vi "Close Session.vi"(8 "error in":errorcluster, 11 "session":refnum<class "Session.lvclass">) -> (0 "error out":errorcluster)   [LabVIEW 2024, in "lib_NI_Advanced HTTP Client.lvlib" / "Session.lvclass"]
doc: "Closes the HTTP client session and deletes all stored cookies, authentication credentials, and HTTP headers associated with the client session. This VI also terminates all HTTP connections and logs out of any authentication, if applicable."
uses:
  Session.lvclass
  Session.lvclass/Session.ctl
  lvwebclient_64.dll
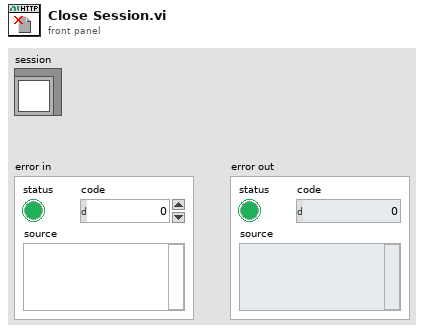
[diagram p1: front panel]
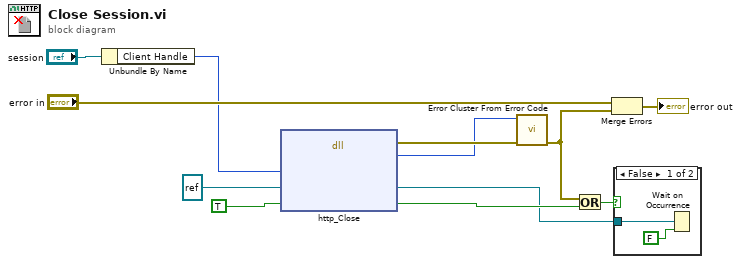
[diagram p0: block diagram]
diagram:
  n1 = Unbundle By Name("session") -> ("Client Handle"=w9:u32)
  n2 = dll-call lib="C:/Program Files/National Instruments/LabVIEW 2024/vi.lib/NI/Advanced HTTP Client/lvwebclient_*.*" fn="http_Close"("handle"=w9, "completeOccurrence"=refnum<k4> refnum ("occurrence"), "closed"=TRUE) -> (error out=w12:errorcluster, "return"=w8:i32, "completeOccurrence"=w1:refnum<k4>, "closed"=w5:bool)  [unwired: 4 in, 1 out]
  n3 = call "Error Cluster From Error Code.vi"("error in (no error)"=w12, "error code (0)"=w8) -> ("error out"=w4:errorcluster)  [unwired: 7 in]
  n4 = Or(x=w4, y=w5) -> (x .or. y?=w2:bool)
  n5 = Merge Errors("error in", w4) -> (→"error out":errorcluster)
  n6 = case shown="False" w2 {
    tunnel: w1 -> [w14 _]
    frame False {
      n7 = Wait on Occurrence(1:FALSE, 2:w14) -> ()  [unwired: 1 in, 1 out]
    }
    frame True {
    }
  }
